vi "Test_ConstructTransport_InvalidRefnum_Error.vi"(8 "error in (no error)":errorcluster, 11 "TestCase in":refnum<class "TestConfigurationFileBinding.lvclass">) -> (0 "error out":errorcluster, 3 "TestCase out":refnum<class "TestConfigurationFileBinding.lvclass">)   [LabVIEW 2017, in "TestConfigurationFileBinding.lvclass"]
uses:
  TestConfigurationFileBinding.lvclass
  <vilib>/Utility/config.llb/Config Data RefNum.ctl
  Source/Concrete/ConfigurationFileBinding/ConfigurationFileBinding.lvclass/ConfigurationFileBinding.ctl
  <vilib>/Utility/error.llb/Error Cluster From Error Code.vi
  <vilib>/Utility/config.llb/Not A Config Data Refnum.vi
  Source/Concrete/ConfigurationFileBinding/ConfigurationFileBinding.lvclass
  <vilib>/Utility/config.llb/NI_LVConfig.lvlib
panel:
  out "Return Error":errorcluster
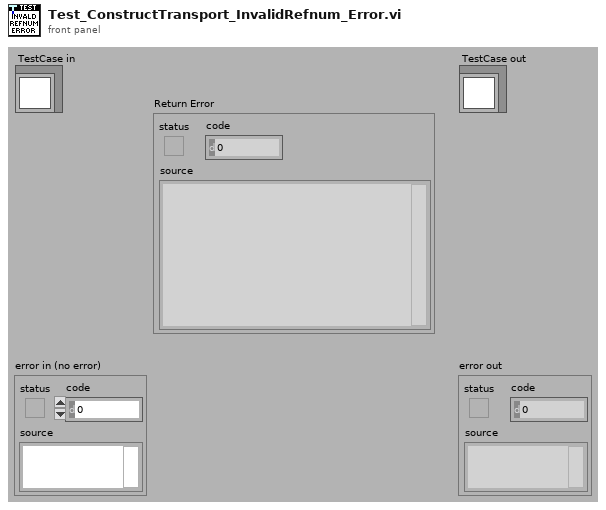
[diagram p1: front panel]
types:
  T1 = typedef "NI_LVConfig.lvlib/Config Data RefNum.ctl" = refnum<k1>
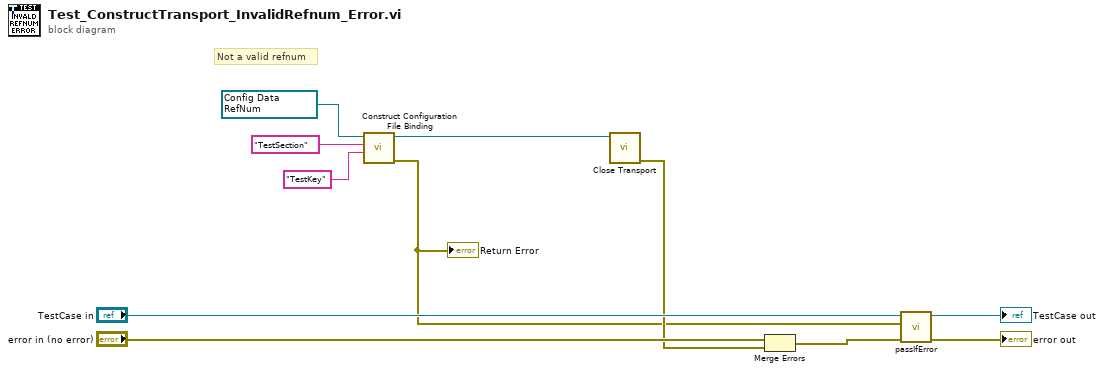
[diagram p0: block diagram]
diagram:
  w2 = T1 refnum items=["config data"] ("Config File Refnum")
  # "Not a valid refnum"
  n1 = call "Construct Configuration File Binding.vi"("Key Name"="TestKey", "Section Name"="TestSection", "Config File Refnum"=w2) -> ("error out"=w1:errorcluster, "ConfigurationFileBinding"=w5:refnum<class "ConfigurationFileBinding.lvclass">)  [unwired: 7 in]
  "Return Error" <- w1
  n2 = call-dynamic "Close Transport.vi"("ITransport in"=w5) -> ("error out"=w3:errorcluster)  [unwired: 10 in]
  n3 = Merge Errors("error in (no error)", w3) -> (w8:errorcluster)
  n4 = call-dynamic "passIfError.vi"("error in (no error)"=w8, "error"=w1, "TestCase in"="TestCase in") -> ("error out"=→"error out":errorcluster, "TestCase out"=→"TestCase out":refnum<class "TestConfigurationFileBinding.lvclass">)  [unwired: 7 in]
